vi "Dequeue.vi"(6 "timeout in ms (-1)":i32=-1, 8 "error in (no error)":errorcluster, 11 "Message Queue":T1) -> (0 "error out":errorcluster, 1 "Message Data":variant, 2 "State":T2, 3 "Message Queue dub":T1, 4 "timed out?":bool, 5 "Call Chain":string[](array[string]))   [LabVIEW 2019, in "Acquire Mouse.lvlib"]
doc: "This VI pulls messages off the Message Queue."
uses:
  Acquire Mouse.lvlib
  State Name.ctl
  Shared/TypeDefs/Message Queue Ref.ctl
  74b75900-f621-4d47-aad2-87bde4252363.vi
  07ac35c6-9def-4c57-8f1c-c738387a4dbe.vi
  <vilib>/Utility/error.llb/Clear Errors.vi
  <vilib>/Utility/error.llb/Error Cluster From Error Code.vi
panel:
  out "# elements in queue":i32
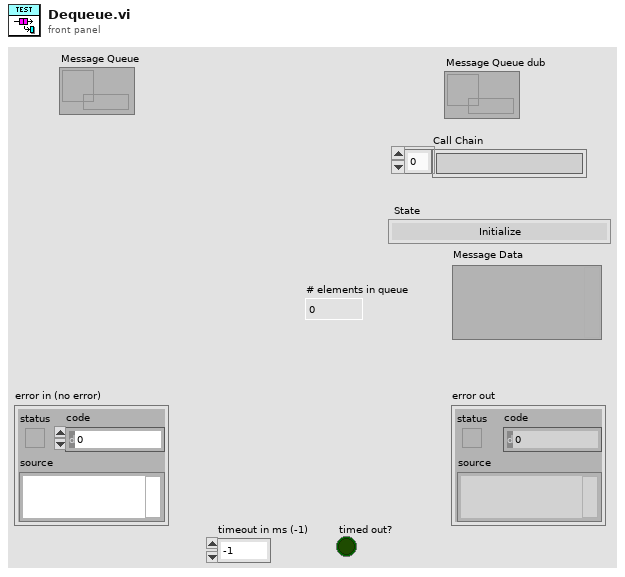
[diagram p1: front panel]
types:
  T1 = typedef "Message Queue Ref.ctl" = refnum<queue>
  T2 = typedef "Acquire Mouse.lvlib/State Name.ctl" = enum16{"Initialize", "Re-Initialize", "Initialize Data", "Initialize Panel", "[Event Structure] Update Data", "Add VI", "Get Splitters", "Map Splitter Pos to Coords", "Initialize Mouse", "Acquire Data", "Process Data", "Error", "Exit", "Default"}
  T3 = cluster{"Custom State Name":string, "Defined State Name":variant, "Call Chain":string[], "Message Data":variant}
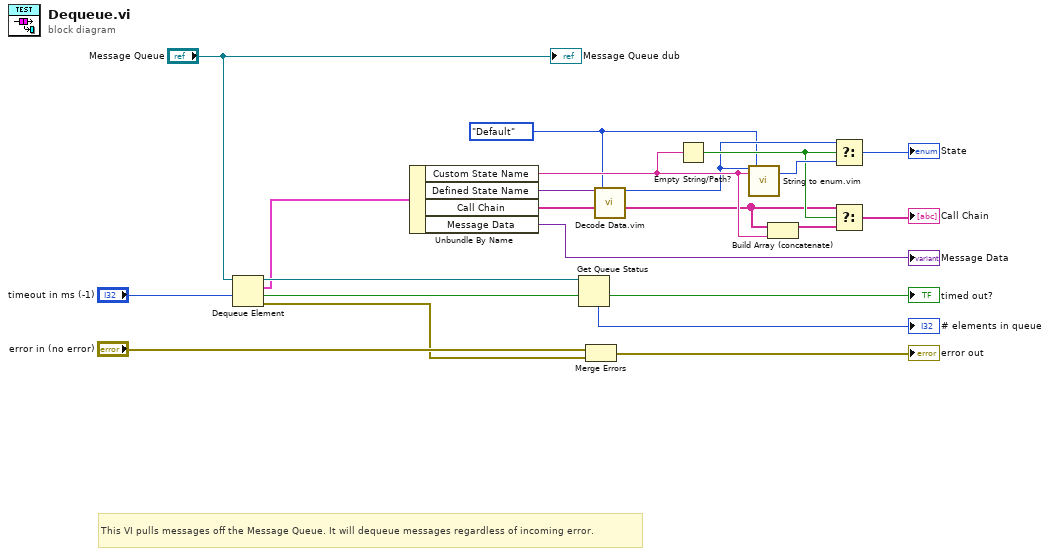
[diagram p0: block diagram]
diagram:
  w5 = State_Name."Default" ("Defined State Name")
  # "This VI pulls messages off the Message Queue. It will dequeue messages regardless of incoming error."
  n1 = Dequeue Element(queue="Message Queue", timeout in ms (-1)="timeout in ms (-1)") -> (queue out=w16:T1, element=w6:T3, timed out?=→"timed out?":bool, error out=w18:errorcluster)  [unwired: 1 in]
  n2 = Unbundle By Name(w6) -> ("Custom State Name"=w9:string, "Defined State Name"=w13:variant, "Call Chain"=w8:string[], "Message Data"=→"Message Data":variant)
  n3 = Get Queue Status(queue=w16) -> (# elements in queue=→"# elements in queue":i32)  [unwired: 2 in, 7 out]
  n4 = Merge Errors("error in (no error)", w18) -> (→"error out":errorcluster)
  n5 = call "Decode Data.vim"("Data"=w13, "Type/Default value"=w5) -> ("Data out"=w7:T2)  [unwired: 16 in, 1 out]
  n6 = Empty String/Path?(string/path=w9) -> (empty?=w11:bool)
  n7 = call "String to enum.vim"("Enum"=w7, "Item Name"=w9, "Default Item Name"=w5) -> ("Enum Selected"=w12:T2)  [unwired: 14 in, 2 out]
  n8 = Build Array (concatenate)(w8, w9) -> (w10:string[])
  n9 = Select(t=w7, s=w11, f=w12) -> (s? t:f=→"State":T2)
  n10 = Select(t=w8, s=w11, f=w10) -> (s? t:f=→"Call Chain":string[])
  "Message Queue dub" <- "Message Queue"
